vi "pl1000CloseUnit.vi"(8 "error in (no error)":errorcluster, 11 "pl1000 handle":i16=16384) -> (0 "error out":errorcluster, 3 "pl1000 handle out":i16)   [LabVIEW 2010]
uses:
  pl1000.dll
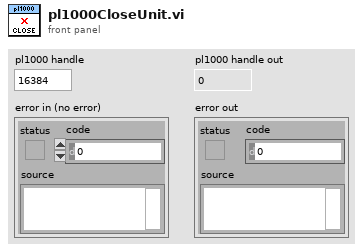
[diagram p1: front panel]
types:
  T1 = cluster{"status":bool, "code":u32, "source":string}
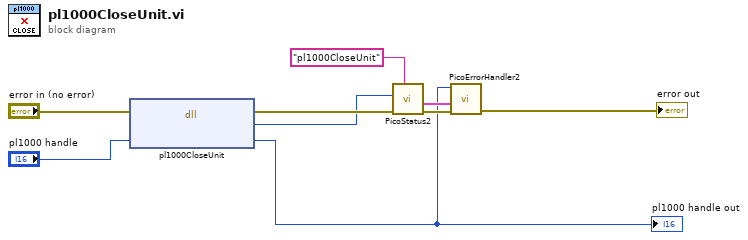
[diagram p0: block diagram]
diagram:
  n1 = dll-call lib="pl1000.dll" fn="pl1000CloseUnit"(error in="error in (no error)", "handle"="pl1000 handle") -> (error out=w5:errorcluster, "status"=w4:u32, "handle"=w3:i16)  [unwired: 2 in, 1 out]
  "pl1000 handle out" <- w3
  n2 = call "PicoStatus2.vi"("PICO source"="pl1000CloseUnit", "Error in"=w5, "PICO STATUS"=w4) -> ("error out"=w7:errorcluster, "PICO_STATUS out"=w6:T1)  [unwired: 5 in]
  n3 = call "PicoErrorHandler2.vi"("error in (no error)"=w7, "PICO_STATUS in"=w6, "handle In"=w3) -> ("error out"=→"error out":errorcluster)  [unwired: 8 in]
